vi "Find Workspace.vi"(8 "Error In":errorcluster, 10 "Control In":T2={"I-O.lvclass"=refnum, "Gantry"=refnum, "Dispenser"="COM1"}, 11 "Carrier Tray in":refnum<class "Assembly Tray.lvclass">) -> (0 "Error Out":errorcluster, 1 "Workspace":T1, 2 "Control Out":T2={"I-O.lvclass"=refnum, "Gantry"=refnum, "Dispenser"="COM1"}, 3 "Carrier Tray Out":refnum<class "Assembly Tray.lvclass">)   [LabVIEW 2021, in "Assembly Tray.lvclass"]
uses:
  Assembly Tray.lvclass
  C:/Users/HEP/Documents/GitHub/UCSB-Gantry-HEP/Classes/Workspace/Fixture.lvclass
  Controller/Controllers.ctl
  Controller/I-O/I-O.lvclass
  C:/Program Files (x86)/Aerotech/A3200/LabVIEW/2010/Bin/Aerotech.A3200.dll
  Program Files (x86)/Aerotech/A3200/LabVIEW/2010/Bin/Aerotech.A3200.dll
  Workspace.ctl
  Fixture.lvclass/Fixture.ctl
  Assembly Tray.lvclass/Assembly Tray.ctl
  Read Fixture ID.vi
  Fixture.lvclass
  Controller/Controller.lvclass
panel:
  out "XYZTheta Centers":dbl[][](array[numeric])
  in  "output cluster 2":T1
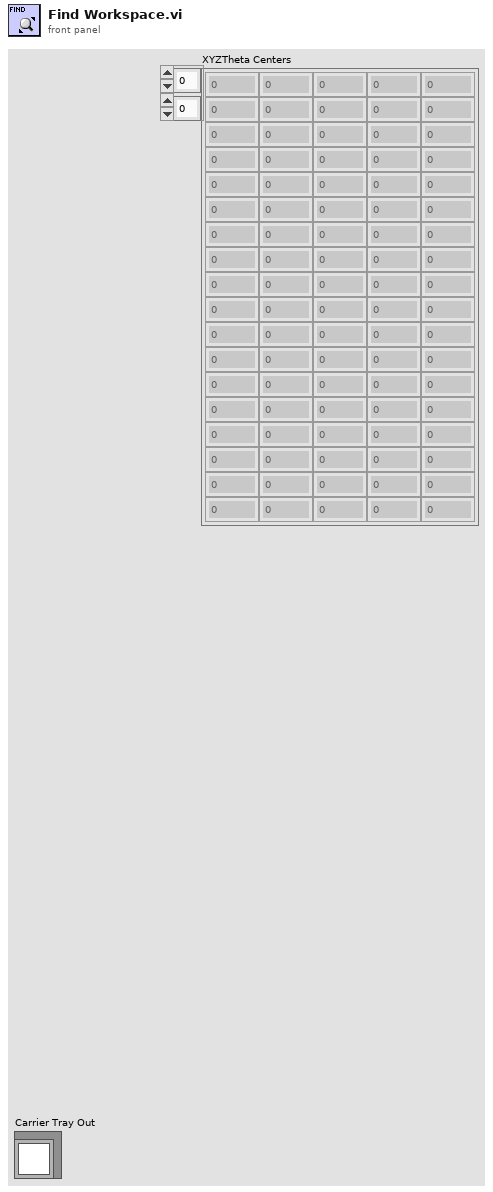
[diagram p1: front panel]
types:
  T1 = typedef "Fixture.lvclass/Workspace.ctl" = cluster{"XYZTheta":dbl[], "Workspace Valve":i32, "Workspace Sensor":i32}
  T2 = typedef "Controller.lvclass/Controllers.ctl" = cluster{"I-O.lvclass":refnum<class "I-O.lvclass">, "Gantry":refnum<k24>, "Dispenser":refnum<visa-resource-name>}
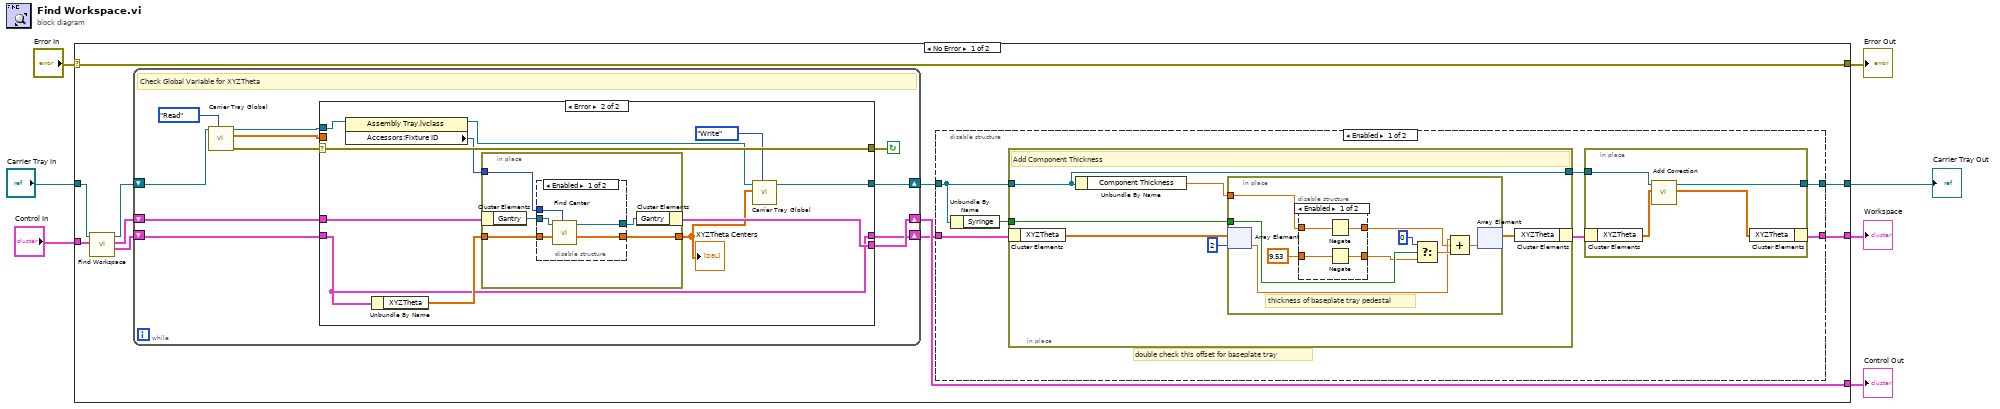
[diagram p0: block diagram]
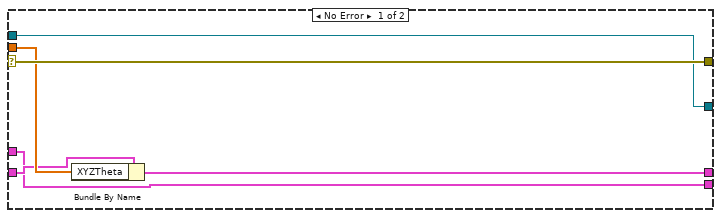
[diagram p4: hidden frame]
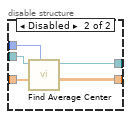
[diagram p5: hidden frame]
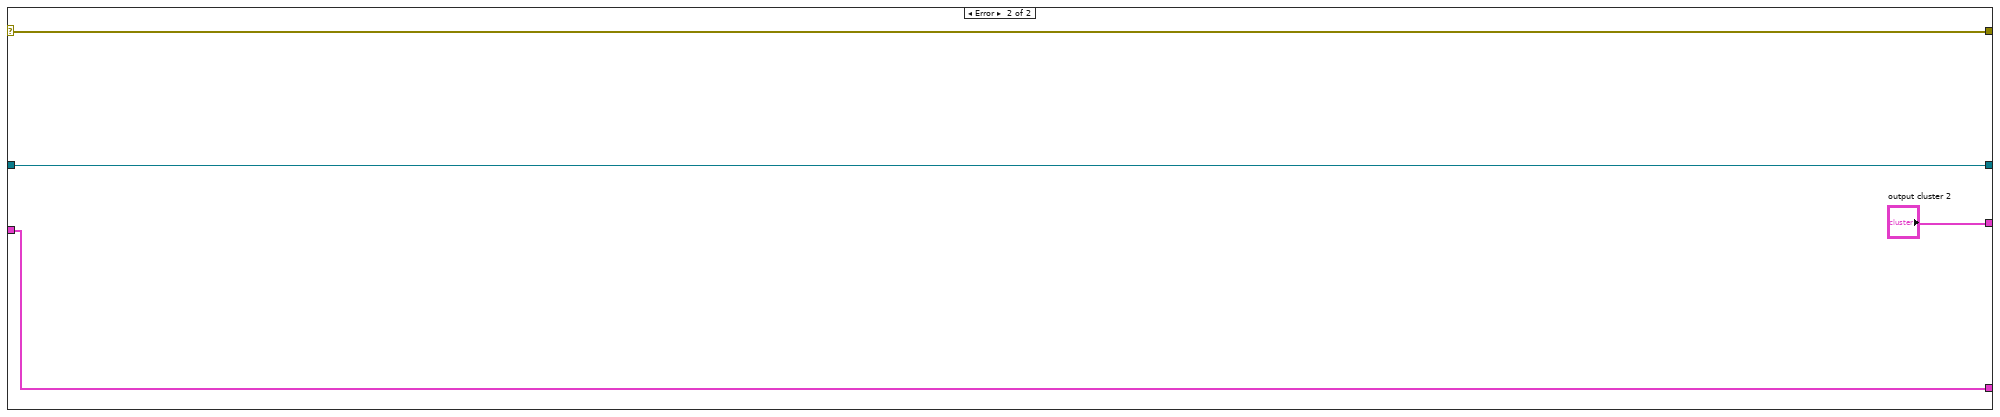
[diagram p6: hidden frame]
diagram:
  n1 = case shown="No Error" "Error In" {
    selector: "Error In" -> [w18 w98]
    tunnel: [w18 w98] -> w6
    tunnel: "Control In" -> [w17 w99]
    tunnel: [w13 w99] -> w4
    tunnel: "Carrier Tray in" -> [w16 w96]
    tunnel: [w14 "output cluster 2"] -> w2
    tunnel: [w15 w96] -> w1
    frame No Error {
      n2 = call-parent "Find Workspace.vi"("Control In"=w17, "Workspace In"=w16) -> (1:"Workspace Out"=w12:T1, "Control Out"=w11:T2, 3:"Workspace Out"=w8:refnum<class "Assembly Tray.lvclass">)  [unwired: 6 in, 1 out]
      n3 = while {
        shift-right: [w56] -> w10
        shift-left: w8 -> [w54]
        shift-right: [w58] -> w13
        shift-left: w11 -> [w59]
        shift-right: [w55] -> w9
        shift-left: w12 -> [w60]
        stop <- w62 continue-if-true
        # "Check Global Variable for XYZTheta"
        n4 = call "Carrier Tray Global.vi"("Action"=enum16{"Initialize", "Read", "Write"}."Read", "Carrier Tray.lvclass"=w54) -> ("error out"=w53:errorcluster, "XYZTheta out"=w61:dbl[], "Carrier Tray.lvclass 2"=w57:refnum<class "Assembly Tray.lvclass">)  [unwired: 7 in]
        n5 = case shown="Error" w53 {
          selector: w53 -> [w69 w80]
          tunnel: [w69 w80] -> w62
          tunnel: w61 -> [w68 _]
          tunnel: [w67 w70] -> w55
          tunnel: w60 -> [w66 w70]
          tunnel: w59 -> [w64 w74]
          tunnel: [w64 w73] -> w58
          tunnel: w57 -> [w65 w77]
          tunnel: [w65 w79] -> w56
          frame No Error {
            n6 = Bundle By Name(cluster=w66, "XYZTheta"=w68) -> (w67:T1)
          }
          frame Error {
            n7 = property class="Assembly Tray.lvclass"(reference=w77) -> (reference out=w76:refnum<class "Assembly Tray.lvclass">, "Accessors:Fixture ID"=w75:i32)  [unwired: 1 in, 1 out]
            n8 = Unbundle By Name(w70) -> ("XYZTheta"=w72:dbl[])
            n9 = in-place {
              in-place-border: w75 -> [w85]
              in-place-border: w72 -> [w82]
              in-place-border: [w81] -> w71
              n10 = in-place-cluster #1(w74) -> ("Gantry"=w84:refnum<k24>)
              n11 = disable-structure shown="Enabled" {
                disable-tunnel: w85 -> [w90 w91]
                disable-tunnel: w84 -> [w89 w95]
                disable-tunnel: [w88 w94] -> w83
                disable-tunnel: w82 -> [w87 w93]
                disable-tunnel: [w86 w92] -> w81
                frame Enabled {
                  n12 = call "Find Center.vi"("Tray Number"=w90, "XYZTheta"=w87, "Gantry In"=w89) -> ("XYZTheta Centers"=w86:dbl[][], "Gantry Out"=w88:refnum<k24>)  [unwired: 7 in]
                }
                frame Disabled {
                  n13 = call "Find Average Center.vi"("Tray Number"=w91, "XYZTheta"=w93, "Gantry In"=w95) -> ("XYZTheta Centers"=w92:dbl[][], "Gantry Out"=w94:refnum<k24>)  [unwired: 7 in]
                }
              }
              n14 = in-place-cluster #1("Gantry"=w83) -> (w73:T2)
            }
            "XYZTheta Centers" <- w71
            n15 = call "Carrier Tray Global.vi"("Action"=enum16{"Initialize", "Read", "Write"}."Write", "XYZTheta in"=w71, "Carrier Tray.lvclass"=w76) -> ("Carrier Tray.lvclass 2"=w79:refnum<class "Assembly Tray.lvclass">)  [unwired: 6 in, 2 out]
          }
        }
      }
      n16 = disable-structure shown="Enabled" {
        disable-tunnel: [w25 w51] -> w15
        disable-tunnel: [w24 w52] -> w14
        disable-tunnel: w10 -> [w23 w51]
        disable-tunnel: w9 -> [w22 w52]
        frame Enabled {
          # "double check this offset for baseplate tray"
          n17 = Unbundle By Name(w23) -> ("Syringe"=w21:bool)
          n18 = in-place {
            in-place-border: w23 -> [w32]
            in-place-border: [w32] -> w20
            in-place-border: w21 -> [w31]
            # "Add Component Thickness"
            n19 = in-place-cluster #2(w22) -> ("XYZTheta"=w30:dbl[])
            n20 = Unbundle By Name(w32) -> ("Component Thickness"=w33:dbl)
            n21 = in-place {
              in-place-border: w33 -> [w39]
              in-place-border: w31 -> [w43]
              # "thickness of baseplate tray pedestal"
              n22 = in-place-array #3(w30, 2) -> (w40:dbl)
              n23 = disable-structure shown="Enabled" {
                disable-tunnel: w39 -> [w48 w50]
                disable-tunnel: [w47 w50] -> w38
                disable-tunnel: 9.53 -> [w46 w49]
                disable-tunnel: [w45 w49] -> w36
                frame Enabled {
                  n24 = Negate(x=w48) -> (-x=w47:dbl)
                  n25 = Negate(x=w46) -> (-x=w45:dbl)
                }
                frame Disabled {
                }
              }
              n26 = Select(t=0, s=w43, f=w36) -> (s? t:f=w41:dbl)
              n27 = Compound Arithmetic op=ADD(w40, w38, w41) -> (w44:dbl)
              n28 = in-place-array #3(w44) -> (w34:dbl[])  [unwired: 1 out]
            }
            n29 = in-place-cluster #2("XYZTheta"=w34) -> (w19:T1)
          }
          n30 = in-place {
            in-place-border: [w29] -> w25
            in-place-border: w20 -> [w28]
            n31 = in-place-cluster #4(w19) -> ("XYZTheta"=w27:dbl[])
            n32 = call "Add Correction.vi"("XYZTheta"=w27, "Carrier Tray in"=w28) -> ("XYZTheta Out"=w26:dbl[], "Carrier Tray out"=w29:refnum<class "Assembly Tray.lvclass">)  [unwired: 7 in, 1 out]
            n33 = in-place-cluster #4("XYZTheta"=w26) -> (w24:T1)
          }
        }
        frame Disabled {
        }
      }
    }
    frame Error {
    }
  }
  "Error Out" <- w6
  "Control Out" <- w4
  "Workspace" <- w2
  "Carrier Tray Out" <- w1
